vi "CalcMzArray.vi"(8 "TrigDelay":dbl, 9 "Sample Rate":dbl, 10 "Depth":i32, 11 "mzCali. (a/b/c)":dbl[](array[numeric])) -> (3 "mzArray":dbl[](array[numeric]))   [LabVIEW 2012]
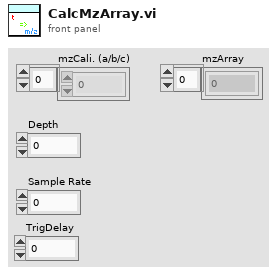
[diagram p1: front panel]
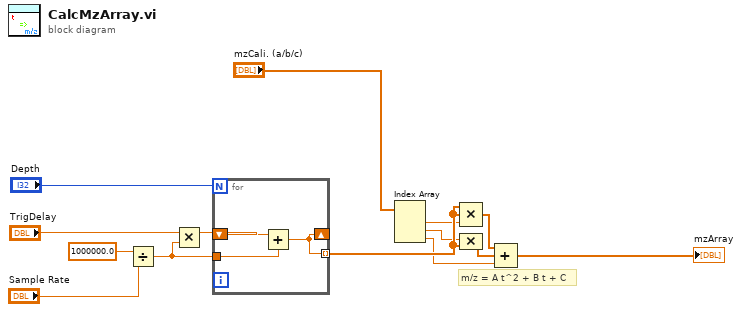
[diagram p0: block diagram]
diagram:
  # "m/z = A t^2 + B t + C"
  n1 = Divide(x=1000000.0, y="Sample Rate") -> (x/y=w1:dbl)
  n2 = Multiply(x="TrigDelay", y=w1) -> (x*y=w2:dbl)
  n3 = for {
    N: "Depth" -> [_]
    shift-right: [w16] -> _
    shift-left: w2 -> [w17]
    tunnel: [w16] -> w10 mode=indexing
    tunnel: w1 -> [w15]
    n4 = Add(x=w17, y=w15) -> (x+y=w16:dbl)
  }
  n5 = Index Array(array="mzCali. (a/b/c)") -> (element #1=w8:dbl, element #2=w7:dbl, element #3=w6:dbl)  [unwired: 3 in]
  n6 = Compound Arithmetic op=MULTIPLY(w10, w10, w8) -> (w4:dbl[])
  n7 = Compound Arithmetic op=MULTIPLY(w7, w10) -> (w5:dbl[])
  n8 = Compound Arithmetic op=ADD(w4, w5, w6) -> (→"mzArray":dbl[])
